vi "Warehouse_Management.vi"() -> ()   [LabVIEW 2015]
uses:
  <vilib>/addons/database/Connection.llb/Conn ObjectReference.ctl
  <vilib>/Utility/miscctls.llb/LVRowAndColumnUnsignedTypeDef.ctl
  Tools/Controls/ITEM_INFORMATION_CLUSTER.ctl
  Tools/Controls/ITEM_CODE_CLUSTER.ctl
  <vilib>/addons/database/Connection.llb/DB Tools Open Connec (Path).vi
  <vilib>/addons/database/Connection.llb/Conn Execute.vi
  <vilib>/addons/database/Recordset.llb/Rec Destroy - Connection.vi
  <vilib>/addons/database/Connection.llb/Conn Get Properties.vi
  <vilib>/addons/database/_DB Variant To Data/Database Variant To Data.xnode
  <vilib>/addons/database/NI_Database_API.lvlib
panel:
  out "connection reference out":T1
  out "CURRENT_YEAR_DATA":string
  in  "INFORMATION_Proccess ready":bool=TRUE
  in  "SUBVI_Proccess ready":bool=TRUE
  out "Find Array":i32[](array[numeric])
  in  "BUTTON_EXIT":bool
  in  "Tab Control":enum32{"Item_Code", "Combo_Box"}(tab)
  in  "TO":timestamp format="%<%d/%m/%Y %H:%M:%S>T"
  in  "FROM":timestamp format="%<%d/%m/%Y %H:%M:%S>T"
  in  "ITEM CODE":string
  in  "Display_Product 2":string caption="Product"
  in  "Display_Part Name 2":string caption="Part Name"
  in  "Display_Maker 2":string caption="Maker"
  in  "Display_Part No. 2":string caption="Part No."
  in  "Display_Lot Size":dbl caption="Lot Size" format="%#_6f"
  in  "Display_Unit":string caption="Unit"
  in  "Display_Location":string caption="Location"
  in  "Next Button":bool
  in  "SEARCH":string
  in  "Combo Box":string(combo)
  in  "Tab Function Control":T2(tab)
  out "INVOICE_ACCESS_TABLE":string[][](table)
  out "INVOICE_STOCK_TABLE":string[][](table)
  out "STORE_ACCESS_TABLE":string[][](table)
  out "STORE_STOCK_TABLE":string[][](table)
  # "INVOICE ACCESS"
  # "INVOICE STOCK"
  # "STORE ACCESS"
  # "STORE STOCK"
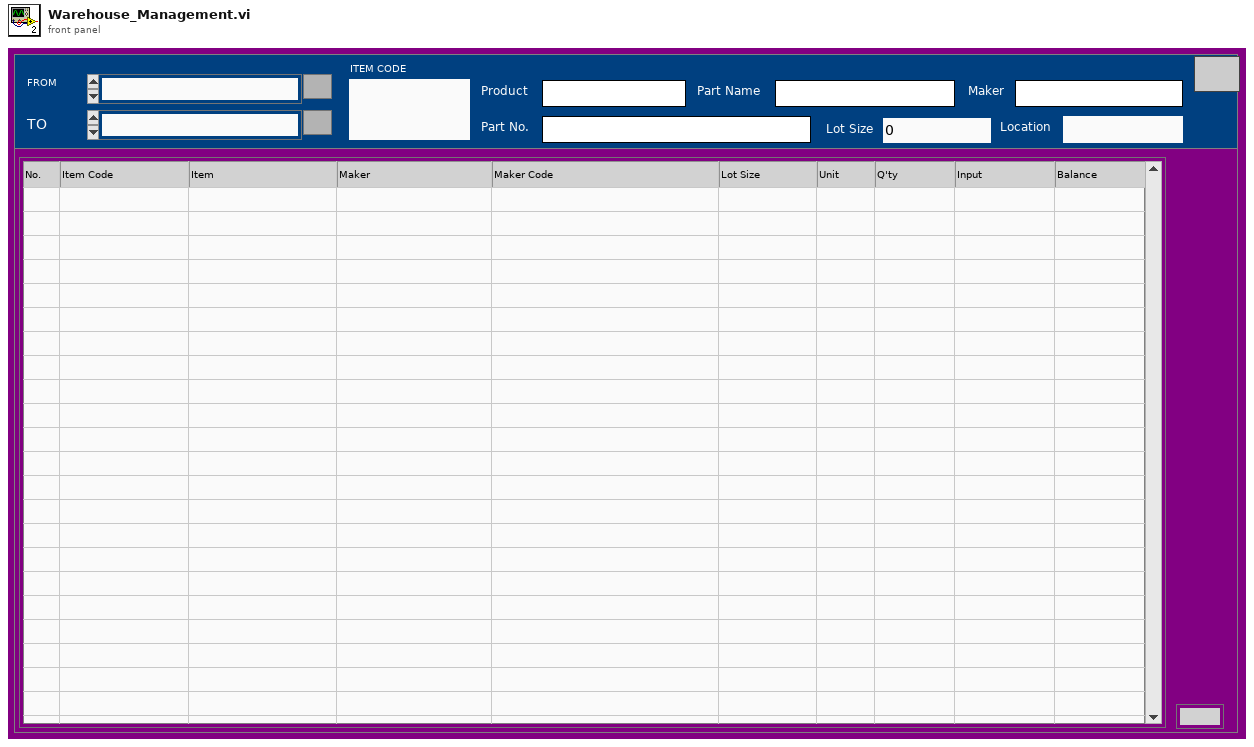
[diagram p1: front panel]
types:
  T1 = typedef "NI_Database_API.lvlib/Conn ObjectReference.ctl" = refnum<k1>
  T2 = enum32{"TAB_INVOICE_ACCESS", "TAB_INVOICE_STOCK", "TAB_STORE_ACCESS", "TAB_STORE_STOCK"}
  T3 = enum16{"open", "replace", "create", "open or create", "replace or create", "replace or create with confirmation"}
  T4 = typedef "LVRowAndColumnUnsignedTypeDef.ctl" = cluster{"Row":u32, "Column":u32}
  T5 = typedef "NI_Database_API.lvlib/Rec ObjectReference.ctl" = refnum<k1>
  T6 = typedef "ITEM_INFORMATION_CLUSTER.ctl" = cluster{"PRODUCT":string, "ITEM_CODE":string, "PART_NAME":string, "MAKER":string, "PART_NO":string, "LOT_SIZE":dbl, "UNIT":string, "LENGTH-OFFSET":string, "BARCODE":string, "PROCESS":string, "INVENTORY_LOCAL":string, "TARE":dbl, "SAMPLE":dbl}
  T7 = typedef "ITEM_CODE_CLUSTER.ctl" = cluster{"ITEM_CODE":string, "INVOICE_NO":string, "INVOICE_DATE":timestamp, "LOT_MAKER":string, "QUANTITY":dbl, "INVOICE_ECODE":string, "INPUT_NO":string, "INPUT_DATE":timestamp, "INPUT_ECODE":string, "LINEBACK_NO":string, "LINEBACK_DATE":timestamp, "LINEBACK_ECODE":string, "OUTPUT_NO":string, "OUTPUT_DATE":timestamp, "OUTPUT_ECODE":string, "DESTINATION":string}
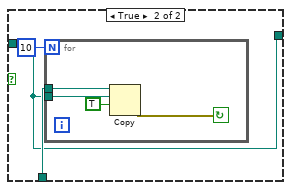
[diagram p3: hidden frame]
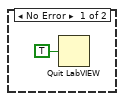
[diagram p7: hidden frame]
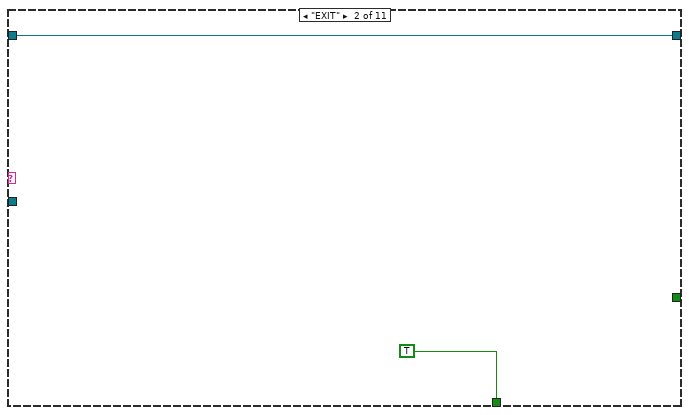
[diagram p10: hidden frame]
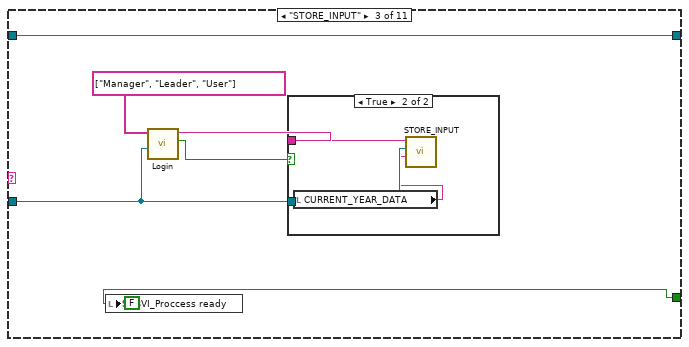
[diagram p11: hidden frame]
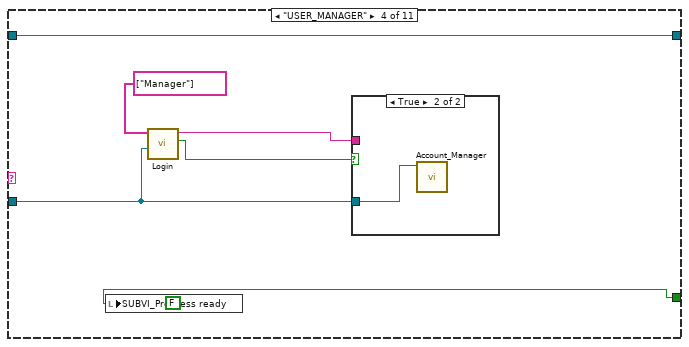
[diagram p13: hidden frame]
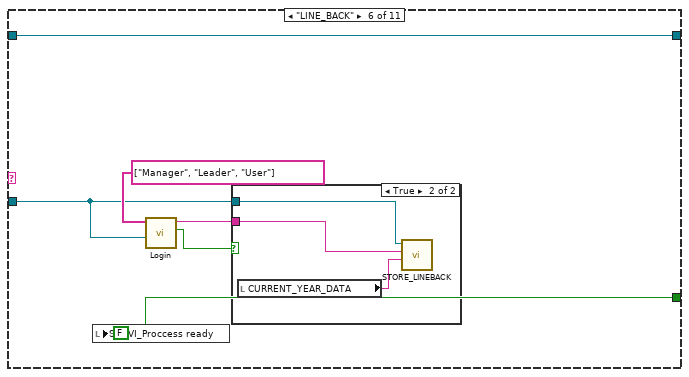
[diagram p16: hidden frame]
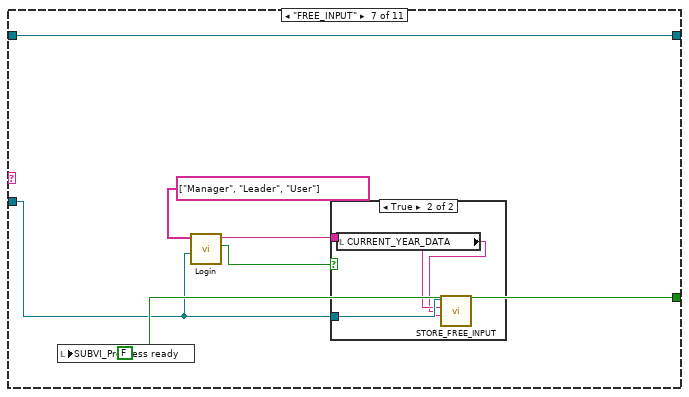
[diagram p18: hidden frame]
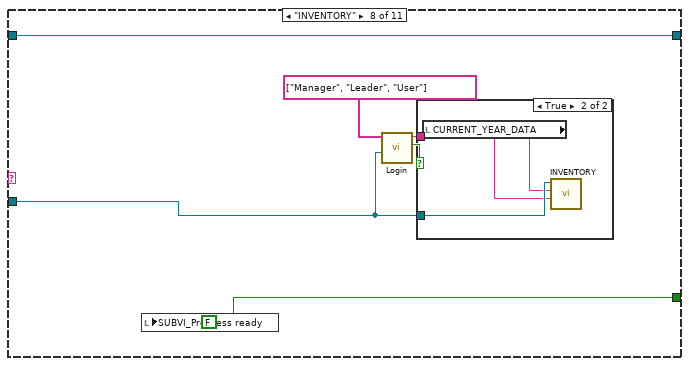
[diagram p20: hidden frame]
diagram:
  n1 = flat-sequence {
    tunnel: [w47] -> w9
    tunnel: [w26] -> w7
    tunnel: [w25] -> w5
    tunnel: [w28] -> w3
    tunnel: [w92] -> w8
    tunnel: w9 -> [w92]
    tunnel: w7 -> [w96]
    tunnel: [w95] -> w6
    tunnel: w5 -> [w95]
    tunnel: [w94] -> w4
    tunnel: w3 -> [w94]
    tunnel: [w93] -> w2
    tunnel: w8 -> [w123]
    tunnel: w6 -> [w122]
    tunnel: w4 -> [w120]
    tunnel: w2 -> [w117]
    frame #0 {
      w60 = "Setting.txt" ("string")
      n2 = call <vilib>:"Application Directory.vi"() -> ("Application Directory"=w66:path)
      n3 = Build Path(base path=w66, name or relative path="setting.txt") -> (appended path=w68:path)
      n4 = Wait (ms)(milliseconds to wait=u32 3000) -> ()  [unwired: 1 out]
      n5 = Open/Create/Replace File(file path (use dialog)=w68, operation (0:open)=T3."open or create", access (0:read/write)=enum16{"read/write", "read-only", "write-only"}."read/write") -> (refnum out=w71:refnum<file>, error out=w72:errorcluster)  [unwired: 3 in, 1 out]
      n6 = Read from Text File(file (use dialog)=w71, error in=w72) -> (refnum out=w73:refnum<file>, text=w61:string, error out=w74:errorcluster)  [unwired: 2 in, 1 out]
      n7 = Match Pattern(string=w61, regular expression="OLD_FILE_NAME>") -> (after substring=w63:string)  [unwired: 1 in, 3 out]
      n8 = Match Pattern(string=w61, regular expression="UPDATE_FILE_NAME>") -> (after substring=w82:string)  [unwired: 1 in, 3 out]
      n9 = Match Pattern(string=w63, regular expression="<") -> ()  [unwired: 1 in, 4 out]
      n10 = Match Pattern(string=w82, regular expression="<") -> ()  [unwired: 1 in, 4 out]
      n11 = Match Pattern(string=w61, regular expression="FILE_NAME>") -> (after substring=w79:string)  [unwired: 1 in, 3 out]
      n12 = Match Pattern(string=w79, regular expression="<") -> ()  [unwired: 1 in, 4 out]
      n13 = Match Pattern(string=w61, regular expression="PATH>") -> (after substring=w76:string)  [unwired: 1 in, 3 out]
      n14 = Close File(refnum=w73, error in=w74) -> ()  [unwired: 2 out]
      n15 = Match Pattern(string=w76, regular expression="<") -> (before substring=w24:string)  [unwired: 1 in, 3 out]
      n16 = String To Path(string=w24) -> (path=w23:path)
      n17 = call <vilib>:"Application Directory.vi"() -> ("Application Directory"=w48:path)
      n18 = Build Path(base path=w48, name or relative path=w60) -> (appended path=w59:path)
      n19 = Build Path(base path=w23, name or relative path=w60) -> (appended path=w58:path)
      n20 = File/Directory Info(path=w59) -> (last mod=w55:timestamp, error out=w54:errorcluster)  [unwired: 1 in, 5 out]
      n21 = File/Directory Info(path=w58) -> (last mod=w56:timestamp, error out=w53:errorcluster)  [unwired: 1 in, 5 out]
      n22 = Or(x=w54, y=w53) -> (x .or. y?=w52:bool)
      n23 = Greater?(x=w56, y=w55) -> (0:w50:bool)
      n24 = Not(x=w52) -> (.not. x?=w51:bool)
      n25 = Select(t=w50, s=w51, f=FALSE) -> (s? t:f=w57:bool)
      n26 = case shown="False" w57 {
        tunnel: w58 -> [_ w87]
        tunnel: w59 -> [w84 w85]
        tunnel: [w84 w85] -> w22
        frame False {
        }
        frame True {
          n27 = for {
            N: 10 -> [_]
            tunnel: w87 -> [w91]
            tunnel: w85 -> [w90]
            stop <- w88 continue-if-true
            n28 = Copy(9:TRUE ("overwrite (F)"), 10:w90, 11:w91) -> (0:w88:errorcluster)  [unwired: 2 in, 2 out]
          }
        }
      }
      n29 = Open/Create/Replace File(file path (use dialog)=w22, operation (0:open)=T3."open or create", access (0:read/write)=enum16{"read/write", "read-only", "write-only"}."read/write") -> (refnum out=w41:refnum<file>, error out=w40:errorcluster)  [unwired: 3 in, 1 out]
      n30 = Read from Text File(file (use dialog)=w41, error in=w40) -> (refnum out=w39:refnum<file>, text=w18:string, error out=w38:errorcluster)  [unwired: 2 in, 1 out]
      n31 = Match Pattern(string=w18, regular expression="OLD_FILE_NAME>") -> (after substring=w45:string)  [unwired: 1 in, 3 out]
      n32 = Match Pattern(string=w18, regular expression="UPDATE_FILE_NAME>") -> (after substring=w30:string)  [unwired: 1 in, 3 out]
      n33 = Match Pattern(string=w45, regular expression="<") -> (before substring=w25:string)  [unwired: 1 in, 3 out]
      n34 = Match Pattern(string=w30, regular expression="<") -> (before substring=w26:string)  [unwired: 1 in, 3 out]
      n35 = Match Pattern(string=w18, regular expression="FILE_NAME>") -> (after substring=w33:string)  [unwired: 1 in, 3 out]
      n36 = Match Pattern(string=w33, regular expression="<") -> (before substring=w28:string)  [unwired: 1 in, 3 out]
      n37 = Match Pattern(string=w18, regular expression="PATH>") -> (after substring=w36:string)  [unwired: 1 in, 3 out]
      n38 = Close File(refnum=w39, error in=w38) -> ()  [unwired: 2 out]
      n39 = Match Pattern(string=w36, regular expression="<") -> (before substring=w27:string)  [unwired: 1 in, 3 out]
      n40 = Match Pattern(string=w18, regular expression="CURRENT_YEAR_DATA>") -> (after substring=w20:string)  [unwired: 1 in, 3 out]
      n41 = Match Pattern(string=w20, regular expression="<") -> ()  [unwired: 1 in, 4 out]
      n42 = String To Path(string=w27) -> (path=w47:path)
    }
    frame #1 {
      n43 = Concatenate Strings(w96, ".exe" ("string")) -> (w93:string)
      n44 = call <vilib>:"Application Directory.vi"() -> ("Application Directory"=w109:path)
      n45 = Build Path(base path=w109, name or relative path=w93) -> (appended path=w98:path)
      n46 = Build Path(base path=w92, name or relative path=w93) -> (appended path=w99:path)
      n47 = File/Directory Info(path=w98) -> (last mod=w102:timestamp, error out=w103:errorcluster)  [unwired: 1 in, 5 out]
      n48 = File/Directory Info(path=w99) -> (last mod=w101:timestamp, error out=w104:errorcluster)  [unwired: 1 in, 5 out]
      n49 = Or(x=w103, y=w104) -> (x .or. y?=w105:bool)
      n50 = Greater?(x=w101, y=w102) -> (0:w107:bool)
      n51 = Not(x=w105) -> (.not. x?=w106:bool)
      n52 = Select(t=w107, s=w106, f=FALSE) -> (s? t:f=w100:bool)
      n53 = case shown="True" w100 {
        tunnel: w99 -> [_ w112]
        tunnel: w98 -> [_ w111]
        frame False {
        }
        frame True {
          n54 = for {
            N: 10 -> [_]
            tunnel: w112 -> [w116]
            tunnel: w111 -> [w115]
            stop <- w113 continue-if-true
            n55 = Copy(9:TRUE ("overwrite (F)"), 10:w115, 11:w116) -> (0:w113:errorcluster)  [unwired: 2 in, 2 out]
          }
        }
      }
    }
    frame #2 {
      w119 = ".exe" ("string")
      n56 = call <vilib>:"Application Directory.vi"() -> ("Application Directory"=w125:path)
      n57 = Concatenate Strings(w120, w119) -> (w118:string)
      n58 = Concatenate Strings(w122, w119) -> (w121:string)
      n59 = Build Path(base path=w125, name or relative path=w121) -> (appended path=w134:path)
      n60 = Build Path(base path=w123, name or relative path=w118) -> (appended path=w135:path)
      n61 = File/Directory Info(path=w134) -> (last mod=w132:timestamp, error out=w131:errorcluster)  [unwired: 1 in, 5 out]
      n62 = File/Directory Info(path=w135) -> (last mod=w133:timestamp, error out=w130:errorcluster)  [unwired: 1 in, 5 out]
      n63 = Or(x=w131, y=w130) -> (x .or. y?=w129:bool)
      n64 = Greater?(x=w133, y=w132) -> (0:w127:bool)
      n65 = Not(x=w129) -> (.not. x?=w128:bool)
      n66 = Select(t=w127, s=w128, f=FALSE) -> (s? t:f=w124:bool)
      n67 = case shown="True" w124 {
        tunnel: w125 -> [_ w141]
        tunnel: w117 -> [_ w136]
        frame False {
        }
        frame True {
          n68 = Two Button Dialog(message="Have an update!\nDo you want to update now?", 1:"No" ("F button name (\"Cancel\")"), 2:"Yes" ("T button name (\"OK\")")) -> (T button?=w137:bool)
          n69 = case shown="True" w137 {
            tunnel: w141 -> [_ w150]
            tunnel: w136 -> [_ w142]
            frame False {
            }
            frame True {
              n70 = Build Path(base path=w150, name or relative path=w142) -> (appended path=w143:path)
              n71 = Format Into String(format string="start \"%s\"", w143) -> (resulting string=w146:string)  [unwired: 2 in, 1 out]
              n72 = Strip Path(path=w143) -> (stripped path=w147:path)  [unwired: 1 out]
              n73 = call <vilib>:"System Exec.vi"("wait until completion? (T)"=FALSE ("Wait until done"), "working directory"=w147, "command line"=w146) -> ("error out"=w148:errorcluster)  [unwired: 5 in, 3 out]
              n74 = case shown="Error" w148 {
                selector: w148 -> [w153 _]
                tunnel: w143 -> [_ w155]
                tunnel: [w153 w154] -> w149
                frame No Error {
                }
                frame Error {
                  # "Win NT/\n2000/XP"
                  n75 = Format Into String(format string="cmd /x /c start \"%s\" \"%s\"", w155, w155) -> (resulting string=w156:string)  [unwired: 2 in, 1 out]
                  n76 = call <vilib>:"System Exec.vi"("wait until completion? (T)"=FALSE ("Wait until done"), "command line"=w156) -> ("error out"=w154:errorcluster)  [unwired: 6 in, 3 out]
                }
              }
              n77 = case shown="Error" w149 {
                frame No Error {
                  n78 = Quit LabVIEW(quit? (T)=TRUE) -> ()
                }
                frame Error {
                  n79 = One Button Dialog(message="Error !\nCan not update ") -> ()  [unwired: 1 in, 1 out]
                }
              }
            }
          }
        }
      }
    }
  }
  n80 = flat-sequence {
    tunnel: [w214] -> w17
    tunnel: [w210] -> w16
    tunnel: [w207] -> w15
    tunnel: [w192] -> w14
    tunnel: ["store_output_information" ("table")] -> w13
    tunnel: [w177] -> w10
    tunnel: [w187] -> w12
    tunnel: [w190] -> w11
    frame #0 {
      w181 = TRUE ("INFORMATION_Proccess ready")
      w190 = "store_INPUT_information" ("table")
      w184 = "warehouse_historydata_%s" ("table")
      w207 = "warehouse_sourcedata" ("table")
      n81 = disable-structure shown="Enabled" {
        disable-tunnel: ["Database" ("userID") w275] -> w203
        frame Disabled {
        }
        frame Enabled {
          n82 = call <vilib>:"Application Directory.vi"() -> ("Application Directory"=w277:path)
          n83 = Build Path(base path=w277, name or relative path="Warehouse_Management.dsn") -> (appended path=w275:path)
        }
      }
      n84 = property on="STORE_ACCESS_TABLE" class="Tbl (strict)"("Index Values"=T4 {"Row"=0, "Column"=0}) -> ()  [unwired: 2 in, 2 out]
      n85 = property on="STORE_STOCK_TABLE" class="Tbl (strict)"("Index Values"=T4 {"Row"=0, "Column"=0}) -> ()  [unwired: 2 in, 2 out]
      n86 = property on="INVOICE_ACCESS_TABLE" class="Tbl (strict)"("Index Values"=T4 {"Row"=0, "Column"=0}) -> ()  [unwired: 2 in, 2 out]
      n87 = local write "BUTTON_EXIT"(FALSE ("BUTTON_EXIT")) -> ()
      n88 = property on="INVOICE_STOCK_TABLE" class="Tbl (strict)"("Index Values"=T4 {"Row"=0, "Column"=0}) -> ()  [unwired: 2 in, 2 out]
      n89 = call-poly <vilib>:"DB Tools Open Connection.vi"("password"="ASTI-WAREHOUSE-PASSWORD" ("name (unnamed)"), "userID"="ASTI-WAREHOUSE", "connection information"=w203) -> ("connection reference"=w199:T1)  [unwired: 5 in, 1 out]
      n90 = local write "SUBVI_Proccess ready"(w181) -> ()
      n91 = local write "INFORMATION_Proccess ready"(w181) -> ()
      n92 = Format Into String(format string="`%s`.`%s`" ("table"), "warehouse_sourcedata" ("table"), "account_information" ("table")) -> (resulting string=w198:string)  [unwired: 2 in, 1 out]
      n93 = call <vilib>:"DB Tools Select Data.vi"("columns"=string[] ["ECODE"], "table"=w198, "connection reference"=w199) -> ("error out"=w197:errorcluster, "connection reference out"=w195:T1)  [unwired: 3 in, 1 out]
      n94 = local write "Tab Function Control"(T2."TAB_STORE_STOCK" ("Tab Function Control")) -> ()
      n95 = local write "Tab Control"(enum32{"Item_Code", "Combo_Box"}."Item_Code" ("Tab Control")) -> ()
      n96 = Format Into String(format string="`%s`.`%s`" ("table"), w207, "item_information" ("table")) -> (resulting string=w192:string)  [unwired: 2 in, 1 out]
      n97 = case shown="Error" w197 {
        tunnel: w195 -> [w312 w313]
        tunnel: w192 -> [_ w325]
        tunnel: [w312 w313] -> w177
        frame No Error {
        }
        frame Error {
          n98 = call-poly <vilib>:"DB Tools Execute Query.vi"("SQL query"="CREATE SCHEMA `warehouse_sourcedata` ;", "connection reference"=w313) -> ("error out"=w334:errorcluster, "recordset reference"=w333:T5)  [unwired: 6 in]
          n99 = call-poly <vilib>:"DB Tools Free Object.vi"("error in (no error)"=w334, "recordset reference"=w333) -> ("error out"=w322:errorcluster, "connection reference"=w332:T1)  [unwired: 8 in]
          n100 = call-poly <vilib>:"DB Tools Execute Query.vi"("SQL query"="\nCREATE TABLE `warehouse_sourcedata`.`account_information` (\n  `ECODE` VARCHAR(20) NOT NULL COMMENT '',\n  `PASSWORD` VARCHAR(45) NULL COMMENT '',\n  `NAME` VARCHAR(45) NULL COMMENT '',\n  `LEVEL` VARCHAR(45) NULL COMMENT '',\n  PRIMARY KEY (`ECODE`)  COMMENT '');", "connection reference"=w332) -> ("error out"=w330:errorcluster, "recordset reference"=w329:T5)  [unwired: 6 in]
          n101 = call-poly <vilib>:"DB Tools Free Object.vi"("error in (no error)"=w330, "recordset reference"=w329) -> ("error out"=w321:errorcluster, "connection reference"=w317:T1)  [unwired: 8 in]
          n102 = Format Into String(format string="CREATE TABLE %s (\n  `PRODUCT` VARCHAR(45) NOT NULL COMMENT '',\n  `ITEM_CODE` VARCHAR(45) NOT NULL COMMENT '',\n  `PART_NAME` VARCHAR(100) NOT NULL COMMENT '',\n  `MAKER` VARCHAR(100)  NULL COMMENT '',\n  `PART_NO` VARCHAR(100)  NULL COMMENT '',\n  `LOT_SIZE` DOUBLE NOT NULL COMMENT '',\n  `UNIT` VARCHAR(20) NULL COMMENT '',\n  `LENGTH-OFFSET` VARCHAR(20) NULL COMMENT '',\n  `BARCODE` VARCHAR(500) NULL COMMENT '',\n  `PROCESS` VARCHAR(100) NULL COMMENT '',\n  `INVENTORY_LOCAL` VARCHAR(100) NULL COMMENT '',\n  `TARE` DOUBLE NULL COMMENT '',\n  `SAMPLE` DOUBLE NULL COMMENT '',\n  PRIMARY KEY (`ITEM_CODE`)  COMMENT '')" ("SQL query"), w325) -> (resulting string=w324:string)  [unwired: 2 in, 1 out]
          n103 = call-poly <vilib>:"DB Tools Execute Query.vi"("SQL query"="CREATE TABLE `warehouse_sourcedata`.`setting_information` (\n  `ID` INT NOT NULL AUTO_INCREMENT,\n  `INFORMATION` VARCHAR(45) NOT NULL,\n  PRIMARY KEY (`ID`));", "connection reference"=w317) -> ("error out"=w318:errorcluster, "recordset reference"=w319:T5)  [unwired: 6 in]
          n104 = call-poly <vilib>:"DB Tools Free Object.vi"("error in (no error)"=w318, "recordset reference"=w319) -> ("error out"=w315:errorcluster, "connection reference"=w316:T1)  [unwired: 8 in]
          n105 = call-poly <vilib>:"DB Tools Execute Query.vi"("SQL query"=w324, "connection reference"=w316) -> ("error out"=w327:errorcluster, "recordset reference"=w328:T5)  [unwired: 6 in]
          n106 = call-poly <vilib>:"DB Tools Free Object.vi"("error in (no error)"=w327, "recordset reference"=w328) -> ("error out"=w320:errorcluster)  [unwired: 8 in, 1 out]
          n107 = Merge Errors(w322, w321, w320, w315) -> (w323:errorcluster)
          n108 = call <vilib>:"Simple Error Handler.vi"("error in (no error)"=w323) -> ()  [unwired: 4 in, 5 out]
        }
      }
      n109 = Obtain Queue(name (unnamed)="SUBVI_Proccess", element data type="", create if not found? (T)=TRUE) -> (queue out=w210:refnum<queue>)  [unwired: 2 in, 2 out]
      n110 = Obtain Queue(name (unnamed)="INFORMATION_Proccess", element data type="", create if not found? (T)=TRUE) -> (queue out=w214:refnum<queue>)  [unwired: 2 in, 2 out]
      n111 = call <vilib>:"DB Tools Select Data.vi"("columns"=string[] ["INFORMATION"], "table"="`warehouse_sourcedata`.`setting_information`", "connection reference"=w177) -> ("data"=w175:variant[][])  [unwired: 3 in, 2 out]
      n112 = xnode "Database Variant To Data"("database variant"=w175, "type"=string[][] []) -> ("data"=w173:string[][])  [unwired: 1 in, 1 out]
      n113 = Index Array(array=w173, index (row)=0 ("index")) -> (element=w169:string[])  [unwired: 1 in]
      n114 = for {
        tunnel: w169 -> [w221] mode=indexing
        tunnel: [w219] -> w168
        stop <- w220 continue-if-true
        n115 = Match Pattern(string=w221, regular expression="CURRENT_YEAR_DATA>") -> (after substring=w223:string)  [unwired: 1 in, 3 out]
        n116 = Match Pattern(string=w223, regular expression="<") -> (before substring=w219:string)  [unwired: 1 in, 3 out]
        n117 = Empty String/Path?(string/path=w219) -> (empty?=w220:bool)
      }
      n118 = Empty String/Path?(string/path=w168) -> (empty?=w171:bool)
      n119 = case shown="True" w171 {
        tunnel: [w225 w226] -> w170
        tunnel: w168 -> [w225 w226]
        frame False {
        }
        frame True {
          n120 = One Button Dialog(message="PLEASE UPDATE CURRENT_YEAR_DATA IN DATABASE !") -> (true=w227:bool)  [unwired: 1 in]
          n121 = disable-structure shown="Enabled" {
            disable-tunnel: w227 -> [w229 _]
            frame Enabled {
              n122 = Quit LabVIEW(quit? (T)=w229) -> ()
            }
            frame Disabled {
            }
          }
        }
      }
      "CURRENT_YEAR_DATA" <- w170
      n123 = Format Into String(format string=w184, w170) -> (resulting string=w187:string)  [unwired: 2 in, 1 out]
      n124 = Decimal String To Number(string=w170) -> (number=w189:i32)  [unwired: 2 in, 1 out]
      n125 = Increment(x=w189) -> (x+1=w188:i32)
      n126 = Number To Decimal String(number=w188) -> (decimal integer string=w183:string)  [unwired: 1 in]
      n127 = Format Into String(format string=w184, w183) -> (resulting string=w178:string)  [unwired: 2 in, 1 out]
      n128 = Format Into String(format string="`%s`.`%s`" ("table"), w178, w190) -> (resulting string=w185:string)  [unwired: 2 in, 1 out]
      n129 = call <vilib>:"DB Tools Select Data.vi"("table"=w185, "connection reference"=w177) -> ("error out"=w194:errorcluster, "connection reference out"=w193:T1)  [unwired: 4 in, 1 out]
      n130 = Build Array(w178, w187) -> (w186:string[])
      n131 = case shown="Error" w194 {
        tunnel: w193 -> [_ w279]
        tunnel: w186 -> [_ w278]
        frame No Error {
        }
        frame Error {
          n132 = for {
            tunnel: w279 -> [w285]
            tunnel: w278 -> [w283] mode=indexing
            n133 = Format Into String(format string="CREATE SCHEMA `%s` ;" ("SQL query"), w283) -> (resulting string=w282:string)  [unwired: 2 in, 1 out]
            n134 = call-poly <vilib>:"DB Tools Execute Query.vi"("SQL query"=w282, "connection reference"=w285) -> ("error out"=w286:errorcluster, "recordset reference"=w287:T5)  [unwired: 6 in]
            n135 = Format Into String(format string="CREATE TABLE `%s`.`store_initail_information` (\n  `DATE` DATETIME NOT NULL COMMENT '',\n `PRODUCT` VARCHAR(50) NULL COMMENT '',\n  `INITAIL_NO` VARCHAR(100) NULL COMMENT '',\n  `ECODE` VARCHAR(45) NULL COMMENT '',\n  PRIMARY KEY (`DATE`)  COMMENT '');\n" ("SQL query"), w283) -> (resulting string=w298:string)  [unwired: 2 in, 1 out]
            n136 = call-poly <vilib>:"DB Tools Free Object.vi"("error in (no error)"=w286, "recordset reference"=w287) -> ("error out"=w281:errorcluster, "connection reference"=w280:T1)  [unwired: 8 in]
            n137 = Format Into String(format string="CREATE TABLE `%s`.`store_input_information` (\n  `INPUT_NO` VARCHAR(200) NOT NULL COMMENT '',\n  `INPUT_DATE` DATETIME NOT NULL COMMENT '',\n  `ECODE` VARCHAR(45) NOT NULL COMMENT '',\n  PRIMARY KEY (  `INPUT_NO`)  COMMENT '');\n", w283) -> (resulting string=w305:string)  [unwired: 2 in, 1 out]
            n138 = Format Into String(format string="CREATE TABLE `%s`.`store_output_information` (\n  `OUTPUT_NO` VARCHAR(200) NOT NULL COMMENT '',\n  `OUTPUT_DATE` DATETIME NOT NULL COMMENT '',\n  `ECODE` VARCHAR(45) NOT NULL COMMENT '',\n  PRIMARY KEY (  `OUTPUT_NO`)  COMMENT '');\n" ("SQL query"), w283) -> (resulting string=w303:string)  [unwired: 2 in, 1 out]
            n139 = Format Into String(format string="CREATE TABLE `%s`.`store_inventory_information` (\n  `DATE` DATETIME NOT NULL COMMENT '',\n  `INVENTORY_NO` VARCHAR(100) NULL COMMENT '',\n  `ECODE` VARCHAR(45) NULL COMMENT '',\n  PRIMARY KEY (`DATE`)  COMMENT '');\n" ("SQL query"), w283) -> (resulting string=w289:string)  [unwired: 2 in, 1 out]
            n140 = call-poly <vilib>:"DB Tools Execute Query.vi"("SQL query"=w305, "connection reference"=w280) -> ("error out"=w311:errorcluster, "recordset reference"=w310:T5)  [unwired: 6 in]
            n141 = call-poly <vilib>:"DB Tools Free Object.vi"("error in (no error)"=w311, "recordset reference"=w310) -> ("error out"=w297:errorcluster, "connection reference"=w309:T1)  [unwired: 8 in]
            n142 = call-poly <vilib>:"DB Tools Execute Query.vi"("SQL query"=w303, "connection reference"=w309) -> ("error out"=w308:errorcluster, "recordset reference"=w307:T5)  [unwired: 6 in]
            n143 = call-poly <vilib>:"DB Tools Free Object.vi"("error in (no error)"=w308, "recordset reference"=w307) -> ("error out"=w296:errorcluster, "connection reference"=w300:T1)  [unwired: 8 in]
            n144 = call-poly <vilib>:"DB Tools Execute Query.vi"("SQL query"=w298, "connection reference"=w300) -> ("error out"=w301:errorcluster, "recordset reference"=w302:T5)  [unwired: 6 in]
            n145 = call-poly <vilib>:"DB Tools Free Object.vi"("error in (no error)"=w301, "recordset reference"=w302) -> ("error out"=w295:errorcluster, "connection reference"=w291:T1)  [unwired: 8 in]
            n146 = call-poly <vilib>:"DB Tools Execute Query.vi"("SQL query"=w289, "connection reference"=w291) -> ("error out"=w293:errorcluster, "recordset reference"=w292:T5)  [unwired: 6 in]
            n147 = call-poly <vilib>:"DB Tools Free Object.vi"("error in (no error)"=w293, "recordset reference"=w292) -> ("error out"=w288:errorcluster)  [unwired: 8 in, 1 out]
            n148 = Merge Errors(w281, w297, w296, w295, w288) -> (w294:errorcluster)
            n149 = call <vilib>:"General Error Handler.vi"("error in (no error)"=w294) -> ()  [unwired: 10 in, 5 out]
          }
        }
      }
      n150 = local write "BUTTON_EXIT"(FALSE ("BUTTON_EXIT")) -> ()
      "STORE_STOCK_TABLE" <- string[][] [["", "", "", "", "", "", "", ""], ["", "", "", "", "", "", "", ""], ["", "", "", "", "", "", "", ""], ["", "", "", "", "", "", "", ""], ["", "", "", "", "", "", "", ""], ["", "", "", "", "", "", "", ""]] ("STORE_STOCK_TABLE")
      "INVOICE_STOCK_TABLE" <- string[][] [] ("INVOICE_STOCK_TABLE")
      "INVOICE_ACCESS_TABLE" <- string[][] [] ("INVOICE_ACCESS_TABLE")
      "STORE_ACCESS_TABLE" <- string[][] [] ("STORE_ACCESS_TABLE")
    }
  }
  n151 = while {
    tunnel: w17 -> [w341]
    tunnel: [w340] -> _
    tunnel: w16 -> [w339]
    tunnel: [w338] -> _
    tunnel: [w337] -> w1
    stop <- w337 stop-if-true
    n152 = event shown="[3] Timeout" {
      selector: _ -> [_ _ _ _ _ _ _ _ _]
      dyn-events: _ -> [_ _ _ _ _ _ _ _ _]
      timeout: -1 -> [_ _ _ _ _ _ _ _ _]
      tunnel: [TRUE _ w359 w403 _ _ _ _ _] -> w337
      tunnel: w341 -> [w349 w357 w362 _ _ w431 w433 w443 w446]
      tunnel: [w348 w356 w360 _ _ w428 w432 w442 w445] -> w340
      tunnel: w339 -> [w347 w354 w363 _ _ _ _ w440 w444]
      tunnel: [w346 w354 w361 _ _ _ _ w440 w444] -> w338
      event "BUTTON_EXIT": Value Change; Panel Close {
        w345 = "EXIT" ("element")
        n153 = event-data() -> ()  [unwired: 1 in, 3 out]
        n154 = Enqueue Element(queue=w349, element=w345) -> (queue out=w348:refnum<queue>, error out=w344:errorcluster)  [unwired: 2 in, 1 out]
        n155 = Enqueue Element(queue=w347, element=w345) -> (queue out=w346:refnum<queue>, error out=w343:errorcluster)  [unwired: 2 in, 1 out]
        n156 = Merge Errors(w343, w344) -> (w342:errorcluster)
        n157 = call <vilib>:"Simple Error Handler.vi"("error in (no error)"=w342) -> ()  [unwired: 4 in, 5 out]
        n158 = local write "BUTTON_EXIT"(TRUE ("BUTTON_EXIT")) -> ()
      }
      event "Combo Box": Value Change; "Combo Box": Mouse Down {
        n159 = event-data() -> ()  [unwired: 1 in, 4 out]
        n160 = local read "INFORMATION_Proccess ready"() -> (w352:bool)
        n161 = case shown="True" w352 {
          tunnel: [_ "COMBO_BOX" ("element")] -> w353
          frame False {
          }
          frame True {
          }
        }
        n162 = Enqueue Element(queue=w357, element=w353) -> (queue out=w356:refnum<queue>, error out=w355:errorcluster)  [unwired: 2 in, 1 out]
        n163 = call <vilib>:"Simple Error Handler.vi"("error in (no error)"=w355) -> ()  [unwired: 4 in, 5 out]
      }
      event Menu Selection (User) {
        n164 = event-data() -> ("ItemTag"=w364:string)  [unwired: 1 in, 6 out]
        n165 = case shown="\"INVOICE_ACCESS\", \"INVOICE_STOCK\", \"PRINT_LABEL\", \"STORE_ACCESS\", \"STORE_STOCK\"" w364 {
          selector: w364 -> [_ w368 _ w387]
          tunnel: w363 -> [w365 w372 w380 w392]
          tunnel: [w365 w371 w378 w392] -> w361
          tunnel: w362 -> [w366 w370 w381 w391]
          tunnel: [w366 w370 w376 w390] -> w360
          tunnel: [_ _ TRUE _] -> w359
          frame "False", Default {
          }
          frame "ADD_ITEM", "CHECK_STOCK", "FREE_INPUT", "IMPORT_ITEM_DATA", "INVENTORY", "LINE_BACK", "STORE_INPUT", "STORE_OUTPUT", "USER_MANAGER" {
            n166 = local read "SUBVI_Proccess ready"() -> (w369:bool)
            n167 = case shown="True" w369 {
              tunnel: w368 -> [_ w374]
              tunnel: [_ w374] -> w367
              frame False {
                n168 = One Button Dialog(message="Please close \"CHECK STOCK\", \"FREE INPUT\", \"INVENTORY\", \"LINE BACK\", \"STORE INPUT\", \"STORE OUTPUT\"") -> ()  [unwired: 1 in, 1 out]
              }
              frame True {
              }
            }
            n169 = Enqueue Element(queue=w372, element=w367) -> (queue out=w371:refnum<queue>)  [unwired: 2 in, 2 out]
          }
          frame "EXIT" {
            w375 = "EXIT" ("element")
            n170 = Enqueue Element(queue=w381, element=w375) -> (queue out=w377:refnum<queue>, error out=w384:errorcluster)  [unwired: 2 in, 1 out]
            n171 = Enqueue Element(queue=w380, element=w375) -> (queue out=w379:refnum<queue>, error out=w383:errorcluster)  [unwired: 2 in, 1 out]
            n172 = Merge Errors(w383, w384) -> (w382:errorcluster)
            n173 = call <vilib>:"Simple Error Handler.vi"("error in (no error)"=w382) -> ()  [unwired: 4 in, 5 out]
            n174 = Enqueue Element(queue=w377, element=w375) -> (queue out=w376:refnum<queue>)  [unwired: 2 in, 2 out]
            n175 = Enqueue Element(queue=w379, element=w375) -> (queue out=w378:refnum<queue>)  [unwired: 2 in, 2 out]
            n176 = local write "BUTTON_EXIT"(TRUE ("BUTTON_EXIT")) -> ()
          }
          frame "INVOICE_ACCESS", "INVOICE_STOCK", "PRINT_LABEL", "STORE_ACCESS", "STORE_STOCK" {
            n177 = local read "INFORMATION_Proccess ready"() -> (w389:bool)
            n178 = case shown="False" w389 {
              tunnel: [_ w394] -> w388
              tunnel: w387 -> [_ w394]
              frame False {
                n179 = One Button Dialog(message="Please close  \"PRINT LABEL\"") -> ()  [unwired: 1 in, 1 out]
              }
              frame True {
              }
            }
            n180 = Enqueue Element(queue=w391, element=w388) -> (queue out=w390:refnum<queue>)  [unwired: 2 in, 2 out]
            n181 = case shown="Default" w387 {
              frame "INVOICE_ACCESS" {
                n182 = local write "Tab Function Control"(T2."TAB_INVOICE_ACCESS" ("Tab Function Control")) -> ()
                n183 = local write "Tab Control"(enum32{"Item_Code", "Combo_Box"}."Combo_Box" ("Tab Control")) -> ()
              }
              frame Default {
              }
              frame "INVOICE_STOCK" {
                n184 = local write "Tab Function Control"(T2."TAB_INVOICE_STOCK" ("Tab Function Control")) -> ()
                n185 = local write "Tab Control"(enum32{"Item_Code", "Combo_Box"}."Item_Code" ("Tab Control")) -> ()
              }
              frame "STORE_ACCESS" {
                n186 = local write "Tab Function Control"(T2."TAB_STORE_ACCESS" ("Tab Function Control")) -> ()
                n187 = local write "Tab Control"(enum32{"Item_Code", "Combo_Box"}."Combo_Box" ("Tab Control")) -> ()
              }
              frame "STORE_STOCK" {
                n188 = local write "Tab Function Control"(T2."TAB_STORE_STOCK" ("Tab Function Control")) -> ()
                n189 = local write "Tab Control"(enum32{"Item_Code", "Combo_Box"}."Item_Code" ("Tab Control")) -> ()
              }
            }
          }
        }
      }
      event Timeout {
        n190 = event-data() -> ()  [unwired: 1 in, 3 out]
        n191 = disable-structure shown="Enabled" {
          disable-tunnel: [w404 _] -> w403
          frame Enabled {
            n192 = for {
              N: 5 -> [_]
              tunnel: [w407] -> w405
              stop <- w407 continue-if-true
              n193 = local read "connection reference out"() -> (w413:T1)
              n194 = Wait (ms)(milliseconds to wait=u32 5000) -> ()  [unwired: 1 out]
              n195 = call-poly <vilib>:"DB Tools Get Properties.vi"("connection reference"=w413) -> ("error out"=w411:errorcluster, "connection reference out"=w412:T1)  [unwired: 4 in, 1 out]
              n196 = case shown="Error" w411 {
                tunnel: w412 -> [w415 w417]
                tunnel: [w415 w416] -> w410
                frame No Error {
                }
                frame Error {
                  n197 = flat-sequence {
                    tunnel: w417 -> [w422]
                    tunnel: [w421] -> w416
                    frame #0 {
                      n198 = disable-structure shown="Enabled" {
                        disable-tunnel: ["Database" ("userID") w424] -> w420
                        frame Disabled {
                        }
                        frame Enabled {
                          n199 = call <vilib>:"Application Directory.vi"() -> ("Application Directory"=w426:path)
                          n200 = Build Path(base path=w426, name or relative path="Warehouse_Management.udl") -> (appended path=w424:path)
                        }
                      }
                      n201 = call <vilib>:"DB Tools Close Connection.vi"("connection reference"=w422) -> ()  [unwired: 6 in, 1 out]
                      n202 = call-poly <vilib>:"DB Tools Open Connection.vi"("password"="871994", "userID"="hoangbao2106", "connection information"=w420) -> ("connection reference"=w421:T1)  [unwired: 5 in, 1 out]
                    }
                  }
                }
              }
              n203 = call-poly <vilib>:"DB Tools Get Properties.vi"("connection reference"=w410) -> ("error out"=w407:errorcluster, "connection reference out"=w409:T1)  [unwired: 4 in, 1 out]
              n204 = local write "connection reference out"(w409) -> ()
              n205 = case shown="Error" w407 {
                frame No Error {
                }
                frame Error {
                  n206 = One Button Dialog(message="Lost Connect!\nTry Again") -> ()  [unwired: 1 in, 1 out]
                }
              }
            }
            n207 = Unbundle By Name(w405) -> ("status"=w404:bool)
          }
          frame Disabled {
          }
        }
      }
      event "ITEM CODE": Mouse Down? {
        n208 = event-data() -> ()  [unwired: 1 in, 8 out]
        n209 = local write "ITEM CODE"("" ("ITEM CODE")) -> ()
        n210 = event-data() -> ()  [unwired: 2 in, 1 out]
      }
      event "SEARCH": Value Change {
        n211 = event-data() -> ()  [unwired: 1 in, 6 out]
        n212 = Enqueue Element(queue=w431, element="SEACHING") -> (queue out=w428:refnum<queue>, error out=w429:errorcluster)  [unwired: 2 in, 1 out]
        n213 = call <vilib>:"Simple Error Handler.vi"("error in (no error)"=w429) -> ()  [unwired: 4 in, 5 out]
      }
      event "Next Button": Value Change {
        n214 = event-data() -> ()  [unwired: 1 in, 6 out]
        n215 = Enqueue Element(queue=w433, element="SEACHING_NEXT") -> (queue out=w432:refnum<queue>, error out=w434:errorcluster)  [unwired: 2 in, 1 out]
        n216 = call <vilib>:"Simple Error Handler.vi"("error in (no error)"=w434) -> ()  [unwired: 4 in, 5 out]
      }
      event "ITEM CODE": Value Change {
        n217 = event-data() -> ("NewVal"=w438:string)  [unwired: 1 in, 5 out]
        n218 = Enqueue Element(queue=w443, element="ITEM_CODE") -> (queue out=w442:refnum<queue>, error out=w441:errorcluster)  [unwired: 2 in, 1 out]
        n219 = Match Pattern(string=w438, regular expression="\\") -> (before substring=w436:string)  [unwired: 1 in, 3 out]
        n220 = call <vilib>:"Simple Error Handler.vi"("error in (no error)"=w441) -> ()  [unwired: 4 in, 5 out]
        n221 = local write "ITEM CODE"(w436) -> ()
      }
      event "FROM", "TO": Value Change; "TO", "FROM": Mouse Down {
        n222 = event-data() -> ()  [unwired: 1 in, 4 out]
        n223 = Enqueue Element(queue=w446, element="ITEM_CODE") -> (queue out=w445:refnum<queue>, error out=w448:errorcluster)  [unwired: 2 in, 1 out]
        n224 = call <vilib>:"Simple Error Handler.vi"("error in (no error)"=w448) -> ()  [unwired: 4 in, 5 out]
      }
    }
  }
  n225 = disable-structure shown="Enabled" {
    disable-tunnel: w1 -> [w449 _]
    frame Enabled {
      n226 = Quit LabVIEW(quit? (T)=w449) -> ()
    }
    frame Disabled {
    }
  }
  n227 = while {
    tunnel: w15 -> [w460]
    tunnel: w14 -> [w459]
    tunnel: w13 -> [w458]
    tunnel: w10 -> [_]
    tunnel: w12 -> [w457]
    tunnel: w11 -> [w456]
    tunnel: w17 -> [w465]
    tunnel: [w463] -> _
    stop <- w451 stop-if-true
    n228 = local read "connection reference out"() -> (w450:T1)
    n229 = Dequeue Element(queue=w465) -> (queue out=w462:refnum<queue>, element=w464:string, error out=w461:errorcluster)  [unwired: 2 in, 1 out]
    n230 = call <vilib>:"Simple Error Handler.vi"("error in (no error)"=w461) -> ()  [unwired: 4 in, 5 out]
    n231 = case shown="\"STORE_STOCK\"" w464 {
      tunnel: [w467 w469 w476 w593 w705 w730 w1154 w1735 w2313 w2380 w2413] -> w463
      tunnel: w462 -> [w467 w469 w476 w593 w707 w731 w1154 w1735 w2313 w2380 w2413]
      tunnel: w460 -> [_ _ _ _ _ _ _ _ _ _ _]
      tunnel: w459 -> [_ _ _ _ _ w726 _ _ _ _ _]
      tunnel: w458 -> [_ _ _ w587 _ _ _ _ _ _ _]
      tunnel: w450 -> [_ _ w475 w592 _ w727 w1153 w1734 _ _ w2408]
      tunnel: w457 -> [_ _ w474 w591 _ _ w1150 w1731 _ _ _]
      tunnel: w456 -> [_ _ w471 _ _ _ _ _ _ _ _]
      tunnel: [_ _ w470 w588 w704 w711 w1149 w1730 w2311 w2379 w2412] -> w454
      tunnel: [TRUE TRUE _ _ _ _ _ _ _ _ _] -> w452
      frame "False", Default {
      }
      frame "EXIT" {
      }
      frame "INVOICE_ACCESS" {
        w470 = FALSE ("INFORMATION_Proccess ready")
        n232 = local read "Combo Box"() -> (w472:string)
        n233 = Empty String/Path?(string/path=w472) -> (empty?=w473:bool)
        n234 = case shown="False" w473 {
          tunnel: w471 -> [_ w542]
          tunnel: w475 -> [w480 w540]
          tunnel: w474 -> [w481 w532]
          tunnel: w472 -> [w479 _]
          frame False {
            n235 = Format Into String(format string="`%s`.`STORE_INPUT_%s`", w481, w479) -> (resulting string=w485:string)  [unwired: 2 in, 1 out]
            n236 = call <vilib>:"DB Tools Select Data.vi"("table"=w485, "connection reference"=w480) -> ("error out"=w478:errorcluster, "data"=w484:variant[][])  [unwired: 4 in, 1 out]
            n237 = xnode "Database Variant To Data"("database variant"=w484, "error in (no error)"=w478, "type"=string[][] []) -> ("data"=w482:string[][], "error out"=w477:errorcluster)
            n238 = local write "INVOICE_ACCESS_TABLE"(w482) -> ()
            n239 = case shown="No Error" w477 {
              frame No Error {
              }
              frame Error {
                n240 = local write "Combo Box"("") -> ()
              }
            }
          }
          frame True {
            n241 = Format Into String(format string="`%s`.`%s`" ("table"), w532, w542) -> (resulting string=w539:string)  [unwired: 2 in, 1 out]
            n242 = call <vilib>:"DB Tools Select Data.vi"("columns"=string[] ["INPUT_NO"], "table"=w539, "connection reference"=w540) -> ("data"=w537:variant[][])  [unwired: 3 in, 2 out]
            n243 = xnode "Database Variant To Data"("database variant"=w537, "type"=string[][] []) -> ("data"=w535:string[][])  [unwired: 1 in, 1 out]
            n244 = Index Array(array=w535, index (col)=0 ("disabled index (col)")) -> (element=w533:string[])  [unwired: 1 in]
            n245 = property on="Combo Box" class="CmbBox"("Strings[]"=w533) -> ()  [unwired: 2 in, 2 out]
          }
        }
        n246 = local write "INFORMATION_Proccess ready"(w470) -> ()
      }
      frame "STORE_ACCESS" {
        w588 = FALSE ("INFORMATION_Proccess ready")
        n247 = local read "Combo Box"() -> (w589:string)
        n248 = Empty String/Path?(string/path=w589) -> (empty?=w590:bool)
        n249 = case shown="False" w590 {
          tunnel: w592 -> [w596 w658]
          tunnel: w591 -> [w598 w650]
          tunnel: w587 -> [_ w649]
          tunnel: w589 -> [w597 _]
          frame False {
            n250 = Format Into String(format string="`%s`.`STORE_OUTPUT_%s`", w598, w597) -> (resulting string=w602:string)  [unwired: 2 in, 1 out]
            n251 = call <vilib>:"DB Tools Select Data.vi"("table"=w602, "connection reference"=w596) -> ("error out"=w595:errorcluster, "data"=w601:variant[][])  [unwired: 4 in, 1 out]
            n252 = xnode "Database Variant To Data"("database variant"=w601, "error in (no error)"=w595, "type"=string[][] []) -> ("data"=w599:string[][], "error out"=w594:errorcluster)
            n253 = case shown="Error" w594 {
              frame No Error {
              }
              frame Error {
                n254 = local write "Combo Box"("" ("Combo Box")) -> ()
              }
            }
            n255 = local write "STORE_ACCESS_TABLE"(w599) -> ()
          }
          frame True {
            n256 = Format Into String(format string="`%s`.`%s`" ("table"), w650, w649) -> (resulting string=w657:string)  [unwired: 2 in, 1 out]
            n257 = call <vilib>:"DB Tools Select Data.vi"("columns"=string[] ["OUTPUT_NO"], "table"=w657, "connection reference"=w658) -> ("data"=w655:variant[][])  [unwired: 3 in, 2 out]
            n258 = xnode "Database Variant To Data"("database variant"=w655, "type"=string[][] []) -> ("data"=w653:string[][])  [unwired: 1 in, 1 out]
            n259 = Index Array(array=w653, index (col)=0 ("disabled index (col)")) -> (element=w651:string[])  [unwired: 1 in]
            n260 = property on="Combo Box" class="CmbBox"("Strings[]"=w651) -> ()  [unwired: 2 in, 2 out]
          }
        }
        n261 = local write "INFORMATION_Proccess ready"(w588) -> ()
      }
      frame "COMBO_BOX" {
        w704 = FALSE ("INFORMATION_Proccess ready")
        n262 = local read "Tab Function Control"() -> (w706:T2)
        n263 = case shown="\"TAB_INVOICE_ACCESS\", Default" w706 {
          tunnel: ["INVOICE_ACCESS" ("element") "STORE_ACCESS" ("element")] -> w708
          frame "TAB_INVOICE_ACCESS", Default {
          }
          frame "TAB_STORE_ACCESS" {
          }
        }
        n264 = Enqueue Element(queue=w707, element=w708) -> (queue out=w705:refnum<queue>)  [unwired: 2 in, 2 out]
        n265 = local write "INFORMATION_Proccess ready"(w704) -> ()
      }
      frame "ITEM_CODE" {
        w711 = FALSE ("INFORMATION_Proccess ready")
        n266 = local read "ITEM CODE"() -> (w724:string)
        n267 = Format Into String(format string="WHERE ITEM_CODE='%s'", w724) -> (resulting string=w723:string)  [unwired: 2 in, 1 out]
        n268 = call <vilib>:"DB Tools Select Data.vi"("condition"=w723, "table"=w726, "connection reference"=w727) -> ("data"=w722:variant[][])  [unwired: 3 in, 2 out]
        n269 = xnode "Database Variant To Data"("database variant"=w722, "type"=T6[] []) -> ("data"=w720:T6[])  [unwired: 1 in, 1 out]
        n270 = Index Array(array=w720, index=0) -> (element=w718:T6)
        n271 = Unbundle By Name(w718) -> ("PRODUCT"=w717:string, "INVENTORY_LOCAL"=w712:string, "PART_NAME"=w715:string, "MAKER"=w714:string, "PART_NO"=w716:string, "LOT_SIZE"=w713:dbl)  [unwired: 3 out]
        n272 = local write "Display_Product 2"(w717) -> ()
        n273 = local write "Display_Part Name 2"(w715) -> ()
        n274 = local write "Display_Part No. 2"(w716) -> ()
        n275 = local write "Display_Maker 2"(w714) -> ()
        n276 = local write "Display_Lot Size"(w713) -> ()
        n277 = local write "Display_Location"(w712) -> ()
        n278 = local read "Tab Function Control"() -> (w729:T2)
        n279 = case shown="\"TAB_STORE_STOCK\"" w729 {
          tunnel: ["INVOICE_ACCESS" ("element") "STORE_ACCESS" ("element") "INVOICE_STOCK" ("element") "STORE_STOCK" ("element")] -> w728
          frame "TAB_INVOICE_ACCESS", Default {
          }
          frame "TAB_STORE_ACCESS" {
          }
          frame "TAB_INVOICE_STOCK" {
          }
          frame "TAB_STORE_STOCK" {
          }
        }
        n280 = Enqueue Element(queue=w731, element=w728) -> (queue out=w730:refnum<queue>)  [unwired: 2 in, 2 out]
        n281 = local write "INFORMATION_Proccess ready"(w711) -> ()
      }
      frame "STORE_STOCK" {
        w1149 = FALSE ("INFORMATION_Proccess ready")
        n282 = local read "ITEM CODE"() -> (w1151:string)
        n283 = Empty String/Path?(string/path=w1151) -> (empty?=w1152:bool)
        n284 = case shown="False" w1152 {
          tunnel: w1153 -> [w1171 _]
          tunnel: w1151 -> [w1168 _]
          tunnel: w1150 -> [w1162 _]
          frame False {
            n285 = Format Into String(format string="`%s`.`%s`" ("table"), w1162, w1168) -> (resulting string=w1167:string)  [unwired: 2 in, 1 out]
            n286 = call <vilib>:"DB Tools Select Data.vi"("table"=w1167, "connection reference"=w1171) -> ("data"=w1170:variant[][], "connection reference out"=w1161:T1)  [unwired: 4 in, 1 out]
            n287 = xnode "Database Variant To Data"("database variant"=w1170, "type"=T7[] []) -> ("data"=w1165:T7[])  [unwired: 1 in, 1 out]
            n288 = local read "FROM"() -> (w1160:timestamp)
            n289 = local read "TO"() -> (w1156:timestamp)
            n290 = Get Date/Time In Seconds() -> (seconds since 1Jan1904=w1157:timestamp)
            n291 = Less?(x=w1156, y=timestamp(3345170400 s since 1904-01-01)) -> (x < y?=w1158:bool)
            n292 = Select(t=w1157, s=w1158, f=w1156) -> (s? t:f=w1155:timestamp)
            n293 = call "CHANGE_ITEM2STOCK.vi"("date (to)"=w1155, "date (From)"=w1160, "connection reference"=w1161, "DATABASE"=w1162, "data"=w1165, "Output Type"="STORE_STOCK") -> ("Table Out"=w1164:string[][])  [unwired: 5 in]
            n294 = local write "STORE_STOCK_TABLE"(w1164) -> ()
            n295 = local write "TO"(w1155) -> ()
          }
          frame True {
          }
        }
        n296 = local write "INFORMATION_Proccess ready"(w1149) -> ()
      }
      frame "INVOICE_STOCK" {
        w1730 = FALSE ("INFORMATION_Proccess ready")
        n297 = local read "ITEM CODE"() -> (w1732:string)
        n298 = Empty String/Path?(string/path=w1732) -> (empty?=w1733:bool)
        n299 = case shown="False" w1733 {
          tunnel: w1734 -> [w1752 _]
          tunnel: w1732 -> [w1748 _]
          tunnel: w1731 -> [w1750 _]
          frame False {
            n300 = Format Into String(format string="`%s`.`%s`" ("table"), w1750, w1748) -> (resulting string=w1747:string)  [unwired: 2 in, 1 out]
            n301 = call <vilib>:"DB Tools Select Data.vi"("table"=w1747, "connection reference"=w1752) -> ("data"=w1751:variant[][], "connection reference out"=w1742:T1)  [unwired: 4 in, 1 out]
            n302 = xnode "Database Variant To Data"("database variant"=w1751, "type"=T7[] []) -> ("data"=w1745:T7[])  [unwired: 1 in, 1 out]
            n303 = local read "FROM"() -> (w1741:timestamp)
            n304 = local read "TO"() -> (w1737:timestamp)
            n305 = Get Date/Time In Seconds() -> (seconds since 1Jan1904=w1740:timestamp)
            n306 = Less?(x=w1737, y=timestamp(3345170400 s since 1904-01-01)) -> (x < y?=w1739:bool)
            n307 = Select(t=w1740, s=w1739, f=w1737) -> (s? t:f=w1736:timestamp)
            n308 = call "CHANGE_ITEM2STOCK.vi"("date (to)"=w1736, "date (From)"=w1741, "connection reference"=w1742, "data"=w1745, "Output Type"="INVOICE_STOCK") -> ("Table Out"=w1744:string[][])  [unwired: 6 in]
            n309 = local write "INVOICE_STOCK_TABLE"(w1744) -> ()
            n310 = local write "TO"(w1736) -> ()
          }
          frame True {
          }
        }
        n311 = local write "INFORMATION_Proccess ready"(w1730) -> ()
      }
      frame "SEACHING" {
        w2311 = FALSE ("INFORMATION_Proccess ready")
        n312 = local read "Tab Function Control"() -> (w2312:T2)
        n313 = case shown="\"TAB_INVOICE_ACCESS\", Default" w2312 {
          tunnel: [w2322 _ w2323 _] -> w2315
          frame "TAB_INVOICE_ACCESS", Default {
            n314 = local read "INVOICE_ACCESS_TABLE"() -> (w2322:string[][])
          }
          frame "TAB_INVOICE_STOCK" {
          }
          frame "TAB_STORE_ACCESS" {
            n315 = local read "STORE_ACCESS_TABLE"() -> (w2323:string[][])
          }
          frame "TAB_STORE_STOCK" {
          }
        }
        n316 = local read "SEARCH"() -> (w2314:string)
        n317 = Index Array(array=w2315, index (col)=1 ("disabled index (col)")) -> (element=w2317:string[])  [unwired: 1 in]
        n318 = for {
          tunnel: w2317 -> [w2331] mode=indexing
          tunnel: w2314 -> [w2330]
          shift-right: [w2328] -> w2320
          shift-left: i32[] [] ("Find Array") -> [w2327]
          shift-right: [w2324] -> _
          shift-left: 0 -> [w2325]
          i -> [w2326]
          n319 = Search and Replace String(input string=w2331, search string=w2330, replace string=w2330) -> (number of replacements=w2329:i32)  [unwired: 5 in, 3 out]
          n320 = case shown="0" w2329 {
            tunnel: [w2333 w2336] -> w2328
            tunnel: w2327 -> [w2333 w2338]
            tunnel: w2326 -> [_ w2337]
            tunnel: w2325 -> [w2332 w2335]
            tunnel: [w2332 w2334] -> w2324
            frame 0 {
            }
            frame 1, Default {
              n321 = Insert Into Array(array=w2338, index=w2335, new element=w2337) -> (w2336:i32[])
              n322 = Increment(x=w2335) -> (x+1=w2334:i32)
            }
          }
        }
        n323 = local write "Find Array"(w2320) -> ()
        n324 = Empty Array?(array=w2320) -> (empty?=w2321:bool)
        n325 = case shown="True" w2321 {
          tunnel: w2314 -> [_ w2349]
          tunnel: w2320 -> [w2343 _]
          tunnel: w2315 -> [_ w2348]
          tunnel: w2312 -> [_ w2347]
          tunnel: w2312 -> [w2340 _]
          frame False {
            n326 = Index Array(array=w2343, index=0) -> (element=w2341:i32)
            n327 = Bundle By Name(cluster=T4 {"Row"=0, "Column"=0} ("Index Values"), "Row"=w2341) -> (w2339:T4)
            n328 = case shown="\"TAB_INVOICE_STOCK\", Default" w2340 {
              tunnel: w2339 -> [w2345 _ w2346 _]
              frame "TAB_INVOICE_ACCESS" {
                n329 = property on="INVOICE_ACCESS_TABLE" class="Tbl (strict)"("Index Values"=w2345) -> ()  [unwired: 2 in, 2 out]
              }
              frame "TAB_INVOICE_STOCK", Default {
              }
              frame "TAB_STORE_ACCESS" {
                n330 = property on="STORE_ACCESS_TABLE" class="Tbl (strict)"("Index Values"=w2346) -> ()  [unwired: 2 in, 2 out]
              }
              frame "TAB_STORE_STOCK" {
              }
            }
          }
          frame True {
            n331 = Index Array(array=w2348, index (col)=4 ("disabled index (col)")) -> (element=w2352:string[])  [unwired: 1 in]
            n332 = for {
              tunnel: w2352 -> [w2363] mode=indexing
              tunnel: w2349 -> [w2362]
              shift-right: [w2360] -> w2350
              shift-left: i32[] [] ("Find Array") -> [w2359]
              shift-right: [w2356] -> _
              shift-left: 0 -> [w2357]
              i -> [w2358]
              n333 = Search and Replace String(input string=w2363, search string=w2362, replace string=w2362) -> (number of replacements=w2361:i32)  [unwired: 5 in, 3 out]
              n334 = case shown="1, Default" w2361 {
                tunnel: [w2365 w2368] -> w2360
                tunnel: w2359 -> [w2365 w2370]
                tunnel: w2358 -> [_ w2369]
                tunnel: w2357 -> [w2364 w2367]
                tunnel: [w2364 w2366] -> w2356
                frame 0 {
                }
                frame 1, Default {
                  n335 = Insert Into Array(array=w2370, index=w2367, new element=w2369) -> (w2368:i32[])
                  n336 = Increment(x=w2367) -> (x+1=w2366:i32)
                }
              }
            }
            n337 = local write "Find Array"(w2350) -> ()
            n338 = Empty Array?(array=w2350) -> (empty?=w2351:bool)
            n339 = case shown="False" w2351 {
              tunnel: w2350 -> [w2374 _]
              tunnel: w2347 -> [w2372 _]
              frame False {
                n340 = Index Array(array=w2374, index=0) -> (element=w2373:i32)
                n341 = Bundle By Name(cluster=T4 {"Row"=0, "Column"=0} ("Index Values"), "Row"=w2373) -> (w2371:T4)
                n342 = case shown="\"TAB_INVOICE_ACCESS\", Default" w2372 {
                  tunnel: w2371 -> [w2377 _ w2378 _]
                  frame "TAB_INVOICE_ACCESS", Default {
                    n343 = property on="INVOICE_ACCESS_TABLE" class="Tbl (strict)"("Index Values"=w2377) -> ()  [unwired: 2 in, 2 out]
                  }
                  frame "TAB_INVOICE_STOCK" {
                  }
                  frame "TAB_STORE_ACCESS" {
                    n344 = property on="STORE_ACCESS_TABLE" class="Tbl (strict)"("Index Values"=w2378) -> ()  [unwired: 2 in, 2 out]
                  }
                  frame "TAB_STORE_STOCK" {
                  }
                }
              }
              frame True {
              }
            }
          }
        }
        n345 = local write "INFORMATION_Proccess ready"(w2311) -> ()
      }
      frame "SEACHING_NEXT" {
        w2379 = FALSE ("INFORMATION_Proccess ready")
        n346 = local read "Tab Function Control"() -> (w2382:T2)
        n347 = case shown="\"TAB_STORE_ACCESS\"" w2382 {
          tunnel: [w2390 _ w2391 _] -> w2383
          frame "TAB_INVOICE_ACCESS", Default {
            n348 = property on="INVOICE_ACCESS_TABLE" class="Tbl (strict)"() -> ("Index Values"=w2390:T4)  [unwired: 2 in, 2 out]
          }
          frame "TAB_INVOICE_STOCK" {
          }
          frame "TAB_STORE_ACCESS" {
            n349 = property on="STORE_ACCESS_TABLE" class="Tbl (strict)"() -> ("Index Values"=w2391:T4)  [unwired: 2 in, 2 out]
          }
          frame "TAB_STORE_STOCK" {
          }
        }
        n350 = local write "Next Button"(FALSE ("Next Button")) -> ()
        n351 = local read "Find Array"() -> (w2386:i32[])
        n352 = Unbundle By Name(w2383) -> ("Row"=w2384:u32)
        n353 = Search 1D Array(1D array=w2386, element=w2384) -> (index of element=w2385:i32)  [unwired: 1 in]
        n354 = case shown="1, Default" w2385 {
          selector: w2385 -> [_ w2404]
          tunnel: w2386 -> [w2395 w2403]
          tunnel: [w2392 w2397] -> w2381
          frame -1 {
            n355 = Index Array(array=w2395, index=u32 0 ("Row")) -> (element=w2393:i32)
            n356 = Bundle By Name(cluster=T4 {"Row"=0, "Column"=0} ("Index Values"), "Row"=w2393) -> (w2392:T4)
          }
          frame 1, Default {
            n357 = Array Size(array=w2403) -> (size(s)=w2406:i32)
            n358 = Increment(x=w2404) -> (x+1=w2398:i32)
            n359 = Decrement(x=w2406) -> (x-1=w2407:i32)
            n360 = Equal?(x=w2407, y=w2404) -> (x = y?=w2405:bool)
            n361 = Select(t=0 ("f"), s=w2405, f=w2398) -> (s? t:f=w2402:i32)
            n362 = Index Array(array=w2403, index=w2402) -> (element=w2400:i32)
            n363 = Bundle By Name(cluster=T4 {"Row"=0, "Column"=0} ("Index Values"), "Row"=w2400) -> (w2397:T4)
          }
        }
        n364 = case shown="\"TAB_STORE_ACCESS\"" w2382 {
          tunnel: w2381 -> [w2388 _ w2389 _]
          frame "TAB_INVOICE_ACCESS", Default {
            n365 = property on="INVOICE_ACCESS_TABLE" class="Tbl (strict)"("Index Values"=w2388) -> ()  [unwired: 2 in, 2 out]
          }
          frame "TAB_INVOICE_STOCK" {
          }
          frame "TAB_STORE_ACCESS" {
            n366 = property on="STORE_ACCESS_TABLE" class="Tbl (strict)"("Index Values"=w2389) -> ()  [unwired: 2 in, 2 out]
          }
          frame "TAB_STORE_STOCK" {
          }
        }
        n367 = local write "INFORMATION_Proccess ready"(w2379) -> ()
      }
      frame "PRINT_LABEL" {
        w2412 = FALSE ("INFORMATION_Proccess ready")
        n368 = call "Login.vi"("connection reference"=w2408, "Permission"=string[] ["Manager", "Leader", "User"]) -> ("OK"=w2410:bool, "ACCOUNT:  2"=w2411:string)  [unwired: 8 in]
        n369 = case shown="True" w2410 {
          tunnel: w2408 -> [_ w2416]
          tunnel: w2411 -> [_ w2415]
          frame False {
          }
          frame True {
            n370 = local read "CURRENT_YEAR_DATA"() -> (w2414:string)
            n371 = call "PRINT_LABEL.vi"("CURRENT_YEAR_DATA"=w2414, "ECODE 2"=w2415, "connection reference"=w2416) -> ()  [unwired: 9 in]
          }
        }
        n372 = local write "INFORMATION_Proccess ready"(w2412) -> ()
      }
    }
    n373 = local read "BUTTON_EXIT"() -> (w453:bool)
    n374 = Or(x=w452, y=w453) -> (x .or. y?=w451:bool)
    n375 = Not(x=w454) -> (.not. x?=w455:bool)
    n376 = local write "INFORMATION_Proccess ready"(w455) -> ()
  }
  n377 = while {
    tunnel: w16 -> [w2427]
    tunnel: [w2425] -> _
    tunnel: w10 -> [_]
    stop <- w2419 stop-if-true
    n378 = local read "connection reference out"() -> (w2417:T1)
    n379 = Dequeue Element(queue=w2427) -> (queue out=w2424:refnum<queue>, element=w2426:string, error out=w2423:errorcluster)  [unwired: 2 in, 1 out]
    n380 = call <vilib>:"Simple Error Handler.vi"("error in (no error)"=w2423) -> ()  [unwired: 4 in, 5 out]
    n381 = case shown="\"STORE_OUTPUT\"" w2426 {
      tunnel: [w2428 w2430 w2436 w2445 w2452 w2461 w2470 w2479 w2488 w2497 w2504] -> w2425
      tunnel: w2424 -> [w2428 w2430 w2436 w2445 w2452 w2461 w2470 w2479 w2488 w2497 w2504]
      tunnel: w2417 -> [_ _ w2431 w2440 w2447 w2456 w2465 w2474 w2483 w2492 w2502]
      tunnel: [_ _ w2432 w2441 w2448 w2457 w2466 w2475 w2484 w2493 w2503] -> w2421
      tunnel: [_ TRUE _ _ _ _ _ _ _ _ _] -> w2418
      frame "False", Default {
      }
      frame "EXIT" {
      }
      frame "STORE_INPUT" {
        w2432 = FALSE ("SUBVI_Proccess ready")
        n382 = local write "SUBVI_Proccess ready"(w2432) -> ()
        n383 = call "Login.vi"("connection reference"=w2431, "Permission"=string[] ["Manager", "Leader", "User"]) -> ("OK"=w2434:bool, "ACCOUNT:  2"=w2433:string)  [unwired: 8 in]
        n384 = case shown="True" w2434 {
          tunnel: w2431 -> [_ w2439]
          tunnel: w2433 -> [_ w2438]
          frame False {
          }
          frame True {
            n385 = local read "CURRENT_YEAR_DATA"() -> (w2437:string)
            n386 = call "STORE_INPUT.vi"("CURRENT_YEAR_DATA"=w2437, "connection reference"=w2439, "ECODE 2"=w2438) -> ()  [unwired: 9 in]
          }
        }
      }
      frame "USER_MANAGER" {
        w2441 = FALSE ("SUBVI_Proccess ready")
        n387 = local write "SUBVI_Proccess ready"(w2441) -> ()
        n388 = call "Login.vi"("connection reference"=w2440, "Permission"=string[] ["Manager"]) -> ("OK"=w2443:bool, "ACCOUNT:  2"=w2442:string)  [unwired: 8 in]
        n389 = case shown="True" w2443 {
          tunnel: w2440 -> [_ w2446]
          tunnel: w2442 -> [_ _]
          frame False {
          }
          frame True {
            n390 = call "Account_Manager.vi"("connection reference"=w2446) -> ()  [unwired: 11 in]
          }
        }
      }
      frame "STORE_OUTPUT" {
        w2448 = FALSE ("SUBVI_Proccess ready")
        n391 = local write "SUBVI_Proccess ready"(w2448) -> ()
        n392 = call "Login.vi"("connection reference"=w2447, "Permission"=string[] ["Manager", "Leader", "User"]) -> ("OK"=w2451:bool, "ACCOUNT:  2"=w2449:string)  [unwired: 8 in]
        n393 = case shown="True" w2451 {
          tunnel: w2447 -> [_ w2454]
          tunnel: w2449 -> [_ w2455]
          frame False {
          }
          frame True {
            n394 = local read "CURRENT_YEAR_DATA"() -> (w2453:string)
            n395 = call "STORE_OUTPUT.vi"("CURRENT_YEAR_DATA"=w2453, "ECODE 2"=w2455, "connection reference"=w2454) -> ()  [unwired: 9 in]
          }
        }
      }
      frame "LINE_BACK" {
        w2457 = FALSE ("SUBVI_Proccess ready")
        n396 = local write "SUBVI_Proccess ready"(w2457) -> ()
        n397 = call "Login.vi"("connection reference"=w2456, "Permission"=string[] ["Manager", "Leader", "User"]) -> ("OK"=w2460:bool, "ACCOUNT:  2"=w2458:string)  [unwired: 8 in]
        n398 = case shown="True" w2460 {
          tunnel: w2456 -> [_ w2464]
          tunnel: w2458 -> [_ w2463]
          frame False {
          }
          frame True {
            n399 = local read "CURRENT_YEAR_DATA"() -> (w2462:string)
            n400 = call "STORE_LINEBACK.vi"("CURRENT_YEAR_DATA"=w2462, "ECODE 2"=w2463, "connection reference"=w2464) -> ()  [unwired: 9 in]
          }
        }
      }
      frame "FREE_INPUT" {
        w2466 = FALSE ("SUBVI_Proccess ready")
        n401 = local write "SUBVI_Proccess ready"(w2466) -> ()
        n402 = call "Login.vi"("connection reference"=w2465, "Permission"=string[] ["Manager", "Leader", "User"]) -> ("OK"=w2469:bool, "ACCOUNT:  2"=w2467:string)  [unwired: 8 in]
        n403 = case shown="True" w2469 {
          tunnel: w2467 -> [_ w2472]
          tunnel: w2465 -> [_ w2473]
          frame False {
          }
          frame True {
            n404 = local read "CURRENT_YEAR_DATA"() -> (w2471:string)
            n405 = call "STORE_FREE_INPUT.vi"("CURRENT_YEAR_DATA"=w2471, "ECODE 2"=w2472, "connection reference"=w2473) -> ()  [unwired: 9 in]
          }
        }
      }
      frame "INVENTORY" {
        w2475 = FALSE ("SUBVI_Proccess ready")
        n406 = local write "SUBVI_Proccess ready"(w2475) -> ()
        n407 = call "Login.vi"("connection reference"=w2474, "Permission"=string[] ["Manager", "Leader", "User"]) -> ("OK"=w2478:bool, "ACCOUNT:  2"=w2476:string)  [unwired: 8 in]
        n408 = case shown="True" w2478 {
          tunnel: w2476 -> [_ w2481]
          tunnel: w2474 -> [_ w2482]
          frame False {
          }
          frame True {
            n409 = local read "CURRENT_YEAR_DATA"() -> (w2480:string)
            n410 = call "INVENTORY.vi"("CURRENT_YEAR_DATA"=w2480, "ECODE 2"=w2481, "connection reference"=w2482) -> ()  [unwired: 9 in]
          }
        }
      }
      frame "IMPORT_ITEM_DATA" {
        w2484 = FALSE ("SUBVI_Proccess ready")
        n411 = local write "SUBVI_Proccess ready"(w2484) -> ()
        n412 = call "Login.vi"("connection reference"=w2483, "Permission"=string[] ["Manager"]) -> ("OK"=w2487:bool, "ACCOUNT:  2"=w2485:string)  [unwired: 8 in]
        n413 = case shown="True" w2487 {
          tunnel: w2485 -> [_ _]
          tunnel: w2483 -> [_ w2491]
          frame False {
          }
          frame True {
            n414 = call "Import_Source_Item_Code.vi"("CONTROL Control"=enum32{"IMPRORT", "ADD"}."IMPRORT", "UPDATE ONLY"=FALSE, "connection reference"=w2491) -> ()  [unwired: 9 in]
          }
        }
      }
      frame "ADD_ITEM" {
        w2493 = FALSE ("SUBVI_Proccess ready")
        n415 = local write "SUBVI_Proccess ready"(w2493) -> ()
        n416 = call "Login.vi"("connection reference"=w2492, "Permission"=string[] ["Manager", "Leader"]) -> ("OK"=w2496:bool, "ACCOUNT:  2"=w2494:string)  [unwired: 8 in]
        n417 = case shown="True" w2496 {
          tunnel: w2494 -> [_ _]
          tunnel: w2492 -> [_ w2500]
          frame False {
          }
          frame True {
            n418 = call "Import_Source_Item_Code.vi"("CONTROL Control"=enum32{"IMPRORT", "ADD"}."ADD", "UPDATE ONLY"=FALSE, "connection reference"=w2500) -> ()  [unwired: 9 in]
          }
        }
      }
      frame "CHECK_STOCK" {
        w2503 = FALSE ("SUBVI_Proccess ready")
        n419 = local read "CURRENT_YEAR_DATA"() -> (w2501:string)
        n420 = local write "SUBVI_Proccess ready"(w2503) -> ()
        n421 = call "CHECK_STOCK.vi"("CURRENT_YEAR_DATA"=w2501, "connection reference"=w2502) -> ()  [unwired: 10 in]
      }
    }
    n422 = local read "BUTTON_EXIT"() -> (w2420:bool)
    n423 = Or(x=w2418, y=w2420) -> (x .or. y?=w2419:bool)
    n424 = Not(x=w2421) -> (.not. x?=w2422:bool)
    n425 = local write "SUBVI_Proccess ready"(w2422) -> ()
  }
  "connection reference out" <- w10
